vi "Read Register (Core).vi"(0 "SLSC Remote in":refnum<class "SLSC Remote.lvclass">, 1 "type":enum16{"U8", "U16", "U32", "U64"}(ring), 5 "device":refnum<k21>="$DefaultDevices", 7 "register address":u32 format="%.0x", 11 "error in (no error)":errorcluster) -> (4 "SLSC Remote out":refnum<class "SLSC Remote.lvclass">, 6 "device out":refnum<k21>, 8 "next register address":u32 format="%.0x", 10 "data out":u64 format="%.0x", 15 "error out":errorcluster)   [LabVIEW 2015, in "SLSC Remote.lvclass"]
uses:
  SLSC Remote.lvclass
  <vilib>/NI/i3 JSON/JSON Generation/Create Value Files/Create Value - Object.vi
  <vilib>/NI/i3 JSON/JSON Generation/Add Object Parameter Files/Add Object Parameter - String.vi
  <vilib>/NI/i3 JSON/JSON Generation/Add Object Parameter Files/Add Object Parameter - Numeric.vi
  <vilib>/NI/NI JSONRPC Server Framework/Classes/Server/Format Client Request (Auto-Increment).vi
  <vilib>/httpClient/POSTBuffer.vi
  <vilib>/NI/i3 JSON/JSON Parsing/Get Object Parameter Files/Get Object Parameter - Numeric.vi
  <vilib>/NI/NI JSONRPC Server Framework/Classes/Server/JSONRPC Server.lvclass
  <vilib>/NI/i3 JSON/i3-json.lvlib
  <vilib>/httpClient/LabVIEWHTTPClient.lvlib
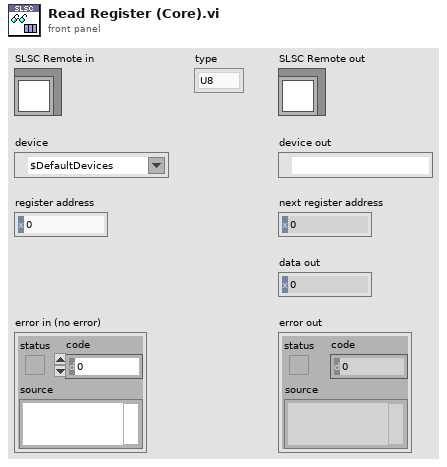
[diagram p1: front panel]
types:
  T1 = typedef "LabVIEWHTTPClient.lvlib/ClientHandle.ctl" = refnum<k1>
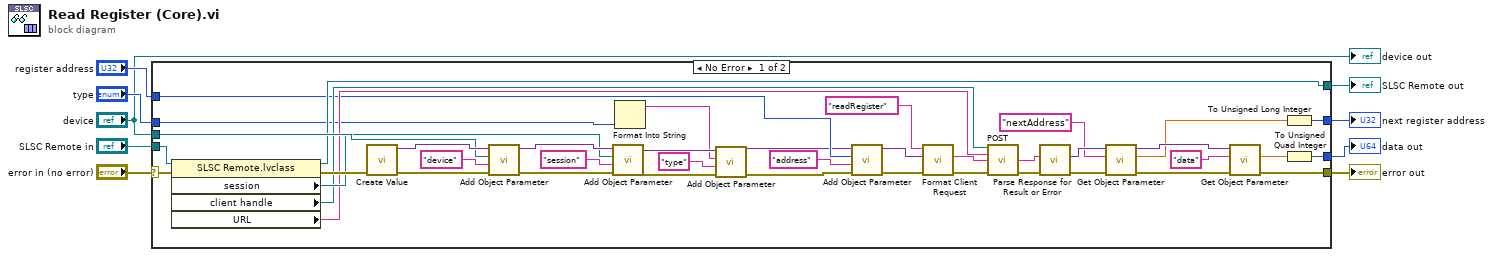
[diagram p0: block diagram]
diagram:
  n1 = case shown="No Error" "error in (no error)" {
    selector: "error in (no error)" -> [w45 w51]
    tunnel: "device" -> [w49 _]
    tunnel: "SLSC Remote in" -> [w47 w52]
    tunnel: [w46 w52] -> w4
    tunnel: [w24 w51] -> w3
    tunnel: "type" -> [w31 _]
    tunnel: "register address" -> [w29 _]
    tunnel: [w20 _] -> w2
    tunnel: [w17 _] -> w1
    frame No Error {
      n2 = property class="SLSC Remote.lvclass"(reference=w47, error in=w45) -> (reference out=w46:refnum<class "SLSC Remote.lvclass">, error out=w44:errorcluster, "session"=w38:refnum<k21>, "client handle"=w36:T1, "URL"=w35:string)
      n3 = call-poly <vilib>:"Create Value.vi"("error in (no error)"=w44) -> ("error out"=w43:errorcluster, "JSON Tree"=w50:variant)  [unwired: 9 in]
      n4 = call-poly <vilib>:"Add Object Parameter.vi"("error in (no error)"=w43, "Name"="device", "String"=w49, "JSON Tree in (JSON Object)"=w50) -> ("error out"=w42:errorcluster, "JSON Tree out (JSON Object)"=w39:variant)  [unwired: 6 in]
      n5 = call-poly <vilib>:"Add Object Parameter.vi"("error in (no error)"=w42, "Name"="session", "String"=w38, "JSON Tree in (JSON Object)"=w39) -> ("error out"=w13:errorcluster, "JSON Tree out (JSON Object)"=w14:variant)  [unwired: 6 in]
      n6 = Format Into String(w31) -> (resulting string=w10:string)  [unwired: 3 in, 1 out]
      n7 = call-poly <vilib>:"Add Object Parameter.vi"("error in (no error)"=w13, "Name"="type", "String"=w10, "JSON Tree in (JSON Object)"=w14) -> ("error out"=w11:errorcluster, "JSON Tree out (JSON Object)"=w12:variant)  [unwired: 6 in]
      n8 = call-poly <vilib>:"Add Object Parameter.vi"("error in (no error)"=w11, "Name"="address", "Numeric"=w29, "JSON Tree in (JSON Object)"=w12) -> ("error out"=w27:errorcluster, "JSON Tree out (JSON Object)"=w28:variant)  [unwired: 6 in]
      n9 = call-poly <vilib>:"Format Client Request.vi"("error in (no error)"=w27, "params"=w28, "method"="readRegister") -> ("error out"=w34:errorcluster, "Request String"=w40:string)  [unwired: 7 in]
      n10 = call-poly <vilib>:"POST.vi"("client handle"=w36, "url"=w35, "buffer"=w40, "error in (no error)"=w34) -> ("body"=w33:string, "error out"=w32:errorcluster)  [unwired: 8 in, 2 out]
      n11 = call <vilib>:"Parse Response for Result or Error.vi"("error in"=w32, "Response String In"=w33) -> ("error out"=w26:errorcluster, "Result or Error Data"=w23:variant)  [unwired: 8 in]
      n12 = call-poly <vilib>:"Get Object Parameter.vi"("error in (no error)"=w26, "Parameter Name"="nextAddress", "JSON Tree In (JSON Object)"=w23) -> ("error out"=w25:errorcluster, "Double Value"=w19:dbl, "JSON Tree Out Passthrough"=w22:variant)  [unwired: 5 in, 1 out]
      n13 = call-poly <vilib>:"Get Object Parameter.vi"("error in (no error)"=w25, "Parameter Name"="data", "JSON Tree In (JSON Object)"=w22) -> ("error out"=w24:errorcluster, "Double Value"=w18:dbl)  [unwired: 5 in, 2 out]
      n14 = To Unsigned Long Integer(number=w19) -> (unsigned 32bit integer=w20:u32)
      n15 = To Unsigned Quad Integer(1:w18) -> (0:w17:u64)
    }
    frame Error {
    }
  }
  "error out" <- w3
  "SLSC Remote out" <- w4
  "next register address" <- w2
  "data out" <- w1
  "device out" <- "device"
